vi "SubVI Translate VHDL.vi"(8 "error in (no error)":errorcluster, 10 "reentrant VIs":string[](array[string]), 11 "SubVI in":refnum<vi>) -> (0 "error out":errorcluster, 1 "reentrant VIs out":string[](array[string]), 2 "transcripted code":string, 3 "transcriptor cluster":T1)   [LabVIEW 2018]
uses:
  types/LabVIEW Universal Transcriptor Cluster.ctl
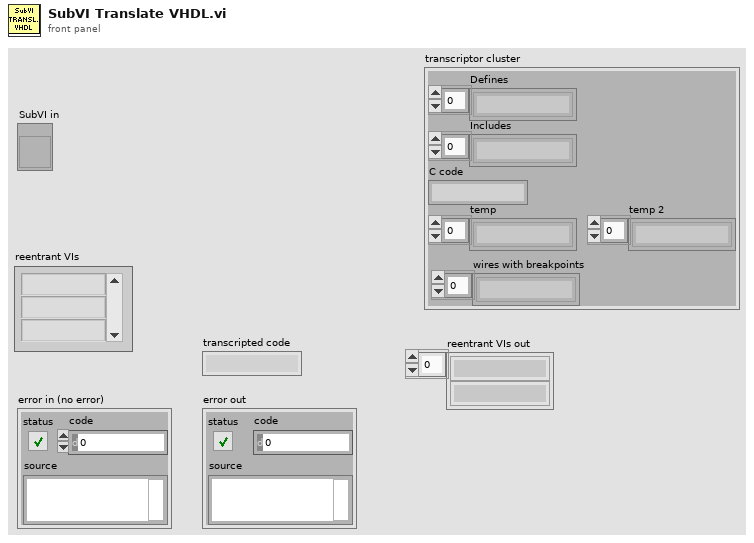
[diagram p1: front panel]
types:
  T1 = typedef "LabVIEW Universal Transcriptor Cluster.ctl" = cluster{"Defines":string[], "Includes":string[], "C code":string, "temp":string[], "temp 2":string[], "wires with breakpoints":string[]}
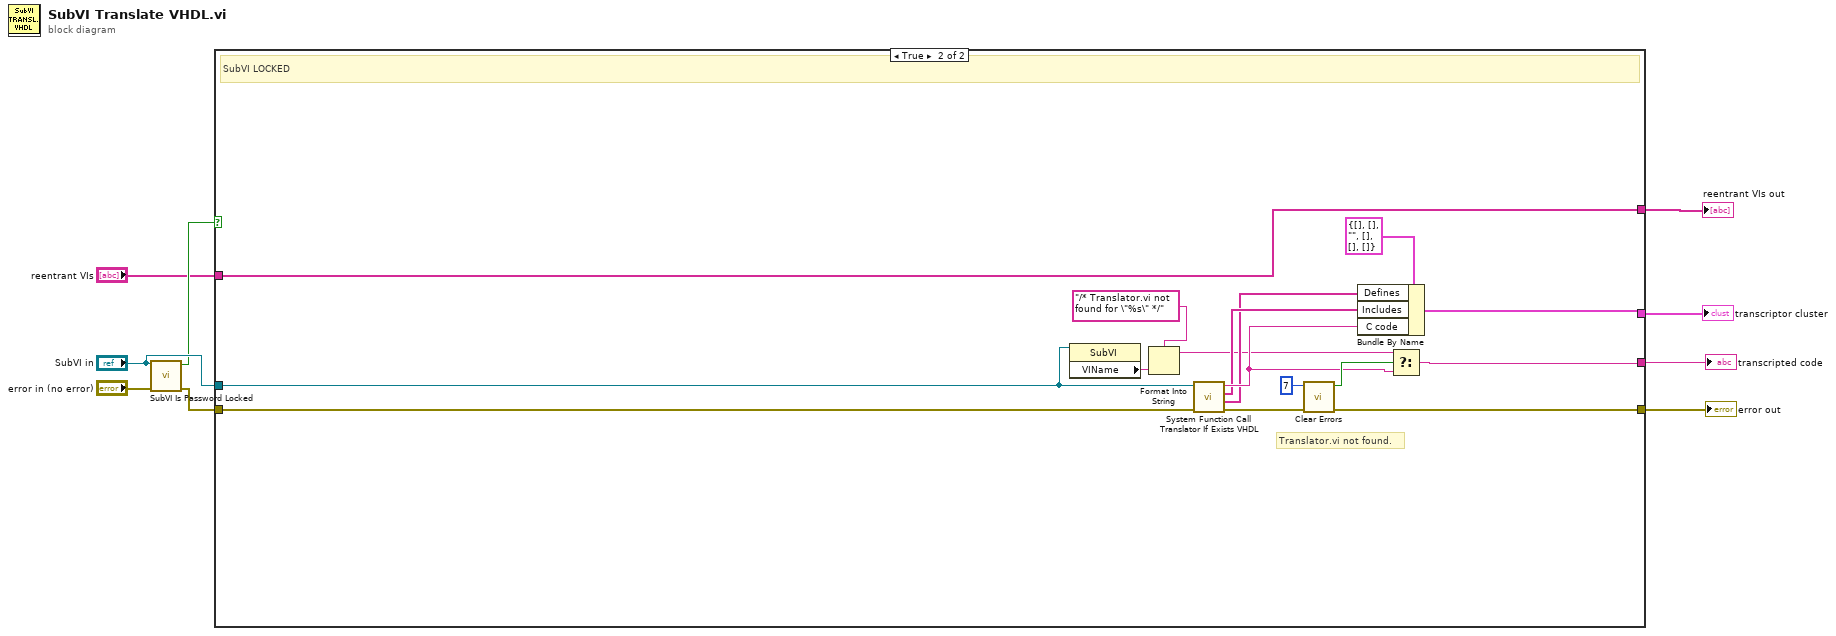
[diagram p0: block diagram]
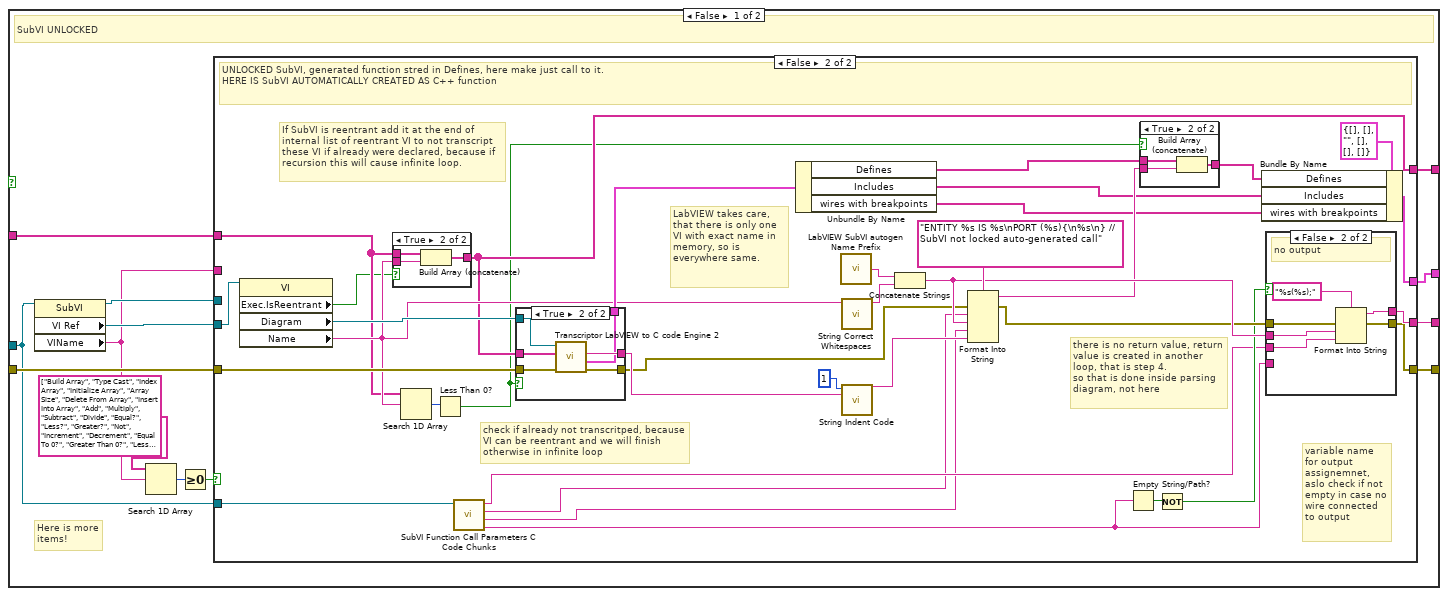
[diagram p2: hidden frame]
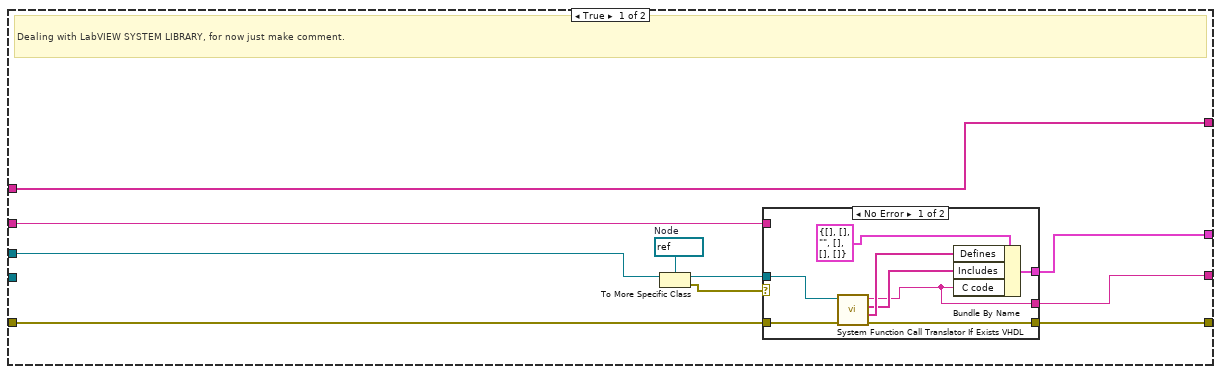
[diagram p3: hidden frame]
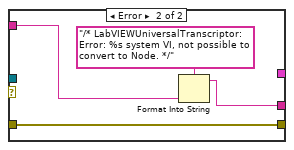
[diagram p4: hidden frame]
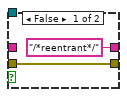
[diagram p7: hidden frame]
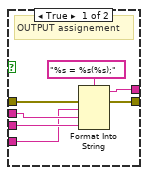
[diagram p8: hidden frame]
diagram:
  n1 = call "SubVI Is Password Locked.vi"("Error In"="error in (no error)", "SubVI ref"="SubVI in") -> ("Error Out"=w8:errorcluster, "isPasswordLocked?"=w5:bool)  [unwired: 8 in]
  n2 = case shown="True" w5 {
    tunnel: "SubVI in" -> [w12 w120]
    tunnel: [w20 w124] -> w7
    tunnel: w8 -> [w22 w123]
    tunnel: [w19 w122] -> w9
    tunnel: [w18 w121] -> w4
    tunnel: "reentrant VIs" -> [w11 w109]
    tunnel: [w10 w109] -> w1
    frame False {
      # "Here is more items!"
      # "SubVI UNLOCKED"
      n3 = property class="SubVI"(reference=w12) -> (reference out=w17:refnum<vi>, "VI Ref"=w21:refnum<vi>, "VIName"=w13:string)  [unwired: 1 in, 1 out]
      n4 = Search 1D Array(1D array=string[] ["Build Array", "Type Cast", "Index Array", "Initialize Array", "Array Size", "Delete From Array", "Insert Into Array", "Add", "Multiply", "Subtract", "Divide", "Equal?", "Less?", "Greater?", "Not", "Increment", "Decrement", "Equal To 0?", "Greater Than 0?", "Less Than 0?", "Greater Or Equal To 0?", "Greater Or Equal?", "Less Or Equal?", "Not Equal?", "Not Equal To 0?", "And", "Or", "Exclusive Or", "To Lower Case", "To Upper Case", "String Length", "String Subset", "Match Pattern", "Decimal String To Number", "Number To Fractional String", "Fract/Exp String To Number", "Number To Decimal String"], element=w13) -> (index of element=w16:i32)  [unwired: 1 in]
      n5 = Greater Or Equal To 0?(x=w16) -> (x >= 0?=w15:bool)
      n6 = case shown="False" w15 {
        tunnel: w22 -> [w30 w54]
        tunnel: w21 -> [_ w66]
        tunnel: [w32 w78] -> w20
        tunnel: [w29 w68] -> w19
        tunnel: w13 -> [w31 _]
        tunnel: [w27 w79] -> w18
        tunnel: w12 -> [_ w64]
        tunnel: w17 -> [w28 _]
        tunnel: w11 -> [w23 w50]
        tunnel: [w23 w49] -> w10
        frame True {
          w26 = refnum<vi> refnum  # Node
          # "Dealing with LabVIEW SYSTEM LIBRARY, for now just make comment."
          n7 = To More Specific Class(target class=w26, reference=w28) -> (specific class reference=w25:refnum<vi>, error out=w24:errorcluster)  [unwired: 1 in]
          n8 = case shown="No Error" w24 {
            tunnel: [w40 w44] -> w29
            tunnel: w25 -> [w39 _]
            tunnel: [w36 _] -> w27
            tunnel: [w35 w41] -> w32
            tunnel: w30 -> [w34 w44]
            tunnel: w31 -> [_ w42]
            frame No Error {
              n9 = call "System Function Call Translator If Exists VHDL.vi"("Error In"=w34, "Node Refnum"=w39) -> ("Error Out"=w40:errorcluster, "Defines"=w38:string[], "Includes"=w37:string[], "Replaced Code"=w35:string)  [unwired: 6 in]
              n10 = Bundle By Name(cluster=T1 {"Defines"=[], "Includes"=[], "C code"="", "temp"=[], "temp 2"=[], "wires with breakpoints"=[]} ("input cluster"), "Defines"=w38, "Includes"=w37, "C code"=w35) -> (w36:T1)
            }
            frame Error {
              n11 = Format Into String(format string="/* LabVIEWUniversalTranscriptor: Error: %s system VI, not possible to convert to Node. */" ("Replaced Code"), w42) -> (resulting string=w41:string)  [unwired: 2 in, 1 out]
            }
          }
        }
        frame False {
          # "If SubVI is reentrant add it at the end of internal list of reentrant VI to not transcript these VI if already were declared, because if recursion this will cause infinite loop."
          # "check if already not transcritped, because VI can be reentrant and we will finish otherwise in infinite loop"
          # "variable name for output assignemnet, aslo check if not empty in case no wire connected to output"
          # "there is no return value, return value is created in another loop, that is step 4.\nso that is done inside parsing diagram, not here"
          # "LabVIEW takes care, that there is only one VI with exact name in memory, so is everywhere same."
          # "UNLOCKED SubVI, generated function stred in Defines, here make just call to it.\nHERE IS SubVI AUTOMATICALLY CREATED AS C++ function"
          n12 = property class="VI"(reference=w66) -> ("Exec.IsReentrant"=w48:bool, "Diagram"=w67:refnum<vi>, "Name"=w51:string)  [unwired: 1 in, 2 out]
          n13 = case shown="True" w48 {
            tunnel: w51 -> [_ w87]
            tunnel: w50 -> [w84 w86]
            tunnel: [w84 w85] -> w49
            frame False {
            }
            frame True {
              n14 = Build Array (concatenate)(w86, w87) -> (w85:string[])
            }
          }
          n15 = Search 1D Array(1D array=w50, element=w51) -> (index of element=w53:i32)  [unwired: 1 in]
          n16 = Less Than 0?(x=w53) -> (x < 0?=w47:bool)
          n17 = call "SubVI Function Call Parameters C Code Chunks.vi"("SubVI Refnum"=w64) -> ("SubVI output variable name"=w62:string, "SubVI func. declaration"=w55:string, "return datatype"=w56:string, "SubVI func. call in code"=w57:string)  [unwired: 5 in, 2 out]
          n18 = case shown="True" w47 {
            tunnel: w54 -> [w89 w95]
            tunnel: [w89 w94] -> w52
            tunnel: ["/*reentrant*/" ("transcripted code") w93] -> w76
            tunnel: w67 -> [_ w92]
            tunnel: [_ w91] -> w60
            tunnel: w49 -> [_ w90]
            frame False {
            }
            frame True {
              n19 = call "Transcriptor LabVIEW to C code Engine 2.vi"("Error In"=w95, "List Reentrant VIs"=w90, "Diagram in"=w92) -> ("error out"=w94:errorcluster, "output cluster"=w91:T1, "transcripted code"=w93:string)  [unwired: 4 in, 2 out]
            }
          }
          n20 = Unbundle By Name(w60) -> ("Defines"=w59:string[], "Includes"=w46:string[], "wires with breakpoints"=w45:string[])
          n21 = call "LabVIEW SubVI autogen Name Prefix.vi"() -> ("datatype prefix"=w74:string)
          n22 = call "String Correct Whitespaces.vi"("String in"=w51) -> ("String out"=w73:string)  [unwired: 10 in]
          n23 = call "String Indent Code.vi"("complete code"=w76, "actual nested level"=1) -> ("indented code"=w65:string)  [unwired: 9 in]
          n24 = Concatenate Strings(w74, w73) -> (w72:string)
          n25 = Format Into String(format string="ENTITY %s IS %s\nPORT (%s){\n%s\n} //SubVI not locked auto-generated call", error in=w52, w56, w72, w55, w65) -> (resulting string=w70:string, error out=w69:errorcluster)  [unwired: 1 in]
          n26 = Empty String/Path?(string/path=w62) -> (empty?=w63:bool)
          n27 = case shown="True" w47 {
            tunnel: [w80 w83] -> w71
            tunnel: w70 -> [_ w82]
            tunnel: w59 -> [w80 w81]
            frame False {
            }
            frame True {
              n28 = Build Array (concatenate)(w81, w82) -> (w83:string[])
            }
          }
          n29 = Not(x=w63) -> (.not. x?=w61:bool)
          n30 = Bundle By Name(cluster=T1 {"Defines"=[], "Includes"=[], "C code"="", "temp"=[], "temp 2"=[], "wires with breakpoints"=[]} ("input cluster"), "Defines"=w71, "Includes"=w46, "wires with breakpoints"=w45) -> (w79:T1)
          n31 = case shown="False" w61 {
            tunnel: [w102 w108] -> w78
            tunnel: w72 -> [w100 w106]
            tunnel: w69 -> [w99 w105]
            tunnel: [w98 w104] -> w68
            tunnel: w57 -> [w97 w103]
            tunnel: w62 -> [w96 _]
            frame True {
              # "OUTPUT assignement"
              n32 = Format Into String(format string="%s = %s(%s);", error in=w99, w96, w100, w97) -> (resulting string=w102:string, error out=w98:errorcluster)  [unwired: 1 in]
            }
            frame False {
              # "no output"
              n33 = Format Into String(format string="%s(%s);", error in=w105, w106, w103) -> (resulting string=w108:string, error out=w104:errorcluster)  [unwired: 1 in]
            }
          }
        }
      }
    }
    frame True {
      # "Translator.vi not found."
      # "SubVI LOCKED"
      n34 = property class="SubVI"(reference=w120) -> ("VIName"=w113:string)  [unwired: 1 in, 2 out]
      n35 = Format Into String(format string="/* Translator.vi not found for \"%s\" */" ("t"), w113) -> (resulting string=w111:string)  [unwired: 2 in, 1 out]
      n36 = call "System Function Call Translator If Exists VHDL.vi"("Error In"=w123, "Node Refnum"=w120) -> ("Error Out"=w119:errorcluster, "Defines"=w114:string[], "Includes"=w115:string[], "Replaced Code"=w116:string)  [unwired: 6 in]
      n37 = call <vilib>:"Clear Errors.vi"("error in (no error)"=w119, "specific error code to clear (0: all)"=7) -> ("error out"=w122:errorcluster, "specific error cleared?"=w117:bool)  [unwired: 4 in]
      n38 = Bundle By Name(cluster=T1 {"Defines"=[], "Includes"=[], "C code"="", "temp"=[], "temp 2"=[], "wires with breakpoints"=[]} ("input cluster"), "Defines"=w114, "Includes"=w115, "C code"=w116) -> (w121:T1)
      n39 = Select(t=w111, s=w117, f=w116) -> (s? t:f=w124:string)
    }
  }
  "error out" <- w9
  "transcripted code" <- w7
  "transcriptor cluster" <- w4
  "reentrant VIs out" <- w1
